vi "LV Image Types.vi"() -> ()   [LabVIEW 2020]
uses:
  <vilib>/picture/picture.llb/imagedata.ctl
panel:
  out "IMAQ Image Display":T1(plugin-control)
  out "Pixmap Image Data":T2
  out "Picture Indicator":picture
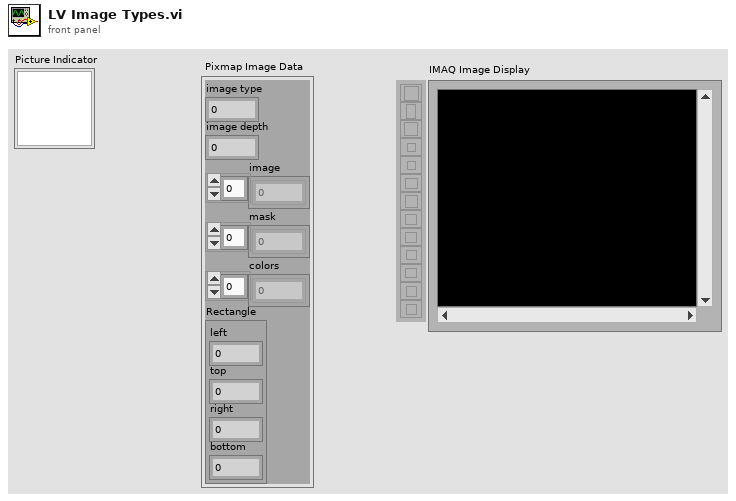
[diagram p1: front panel]
types:
  T1 = typedef "IMAQ Image.ctl" = refnum<image>
  T2 = typedef "imagedata.ctl" = cluster{"image type":i32, "image depth":i32, "image":u8[], "mask":u8[], "colors":u32[], "Rectangle":cluster{"left":i16, "top":i16, "right":i16, "bottom":i16}}
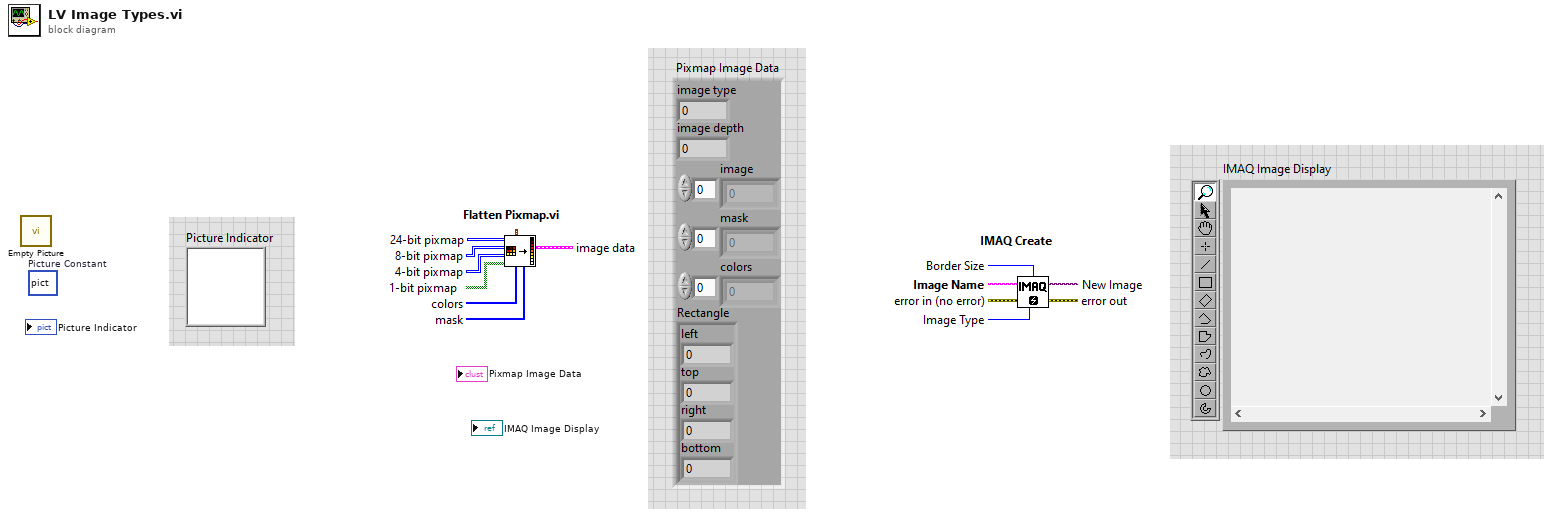
[diagram p0: block diagram]
diagram:
  (unwired) picture data[5B]  # Picture Constant
  n1 = call "Empty Picture"() -> ()  [unwired: 1 out]
